vi "rsidr_core_global.vi"() -> ()   [LabVIEW 2020, in "Rohde&Schwarz RTx Oscilloscopes.lvlib"] (continued)
{"Level"=3, "Class Only"=FALSE, "Identifier"="RSRTX_ATTR_QUICK_MEASUREMENTS_DISABLE", "Descriptive Name"="Quick Measurements Disable", "Data Type"=4, "Command"="MEAS{Measurement}:AOFF", "Access"=1, "Range Table"="", "Read Callback"="", "Write Callback"="", "Supported Models"="", "Instrument Options"="", "Flags"=0, "Help"="Disables all additional measurements in all categories of the indicated measurement.\n\nAvailable Repeated Capabilities:\nMeasurement: M1, M2, M3, M4, M5, M6, M7, M8\r\n\nRemote-control command(s):\nMEASurement<m>:AOFF"}, {"Level"=3, "Class Only"=FALSE, "Identifier"="RSRTX_ATTR_QUICK_MEASUREMENTS_ENABLE_WITH_STATUS_BIT", "Descriptive Name"="Quick Measurements Enable With Status Bit", "Data Type"=3, "Command"="MEAS{Measurement}:ALL", "Access"=2, "Range Table"="", "Read Callback"="", "Write Callback"="", "Supported Models"="", "Instrument Options"="", "Flags"=0, "Help"="Enables and disables quick measurement.\n\nAvailable Repeated Capabilities:\nMeasurement: M1, M2, M3, M4, M5, M6, M7, M8\r\n\nRemote-control command(s):\nMEASurement<m>:ALL[:STATe]"}, {"Level"=2, "Class Only"=TRUE, "Identifier"="", "Descriptive Name"="Automatic Measurements - Statistics", "Data Type"=0, "Command"="", "Access"=0, "Range Table"="", "Read Callback"="", "Write Callback"="", "Supported Models"="", "Instrument Options"="", "Flags"=0, "Help"="Automatic Measurements - Statistics settings and results"}, {"Level"=3, "Class Only"=FALSE, "Identifier"="RSRTX_ATTR_AUTOMATIC_MEASUREMENT_ENABLED", "Descriptive Name"="Automatic Measurement Enabled", "Data Type"=3, "Command"="MEAS{Measurement}:STAT", "Access"=2, "Range Table"="", "Read Callback"="", "Write Callback"="", "Supported Models"="", "Instrument Options"="", "Flags"=0, "Help"="Activates or deactivates the statistical evaluation for the selected measurement.\n\nAvailable Repeated Capabilities:\nMeasurement: M1, M2, M3, M4, M5, M6, M7, M8\r\n\nRemote-control command(s):\nMEASurement<m>:STATistics[:ENABle]"}, {"Level"=3, "Class Only"=FALSE, "Identifier"="RSRTX_ATTR_AUTOMATIC_MEASUREMENT_NUMBER_OF_WAVEFORMS", "Descriptive Name"="Automatic Measurement Number Of Waveforms", "Data Type"=0, "Command"="MEAS{Measurement}:STAT:WEIG?", "Access"=0, "Range Table"="rsrtx_rngAutoMeasWaveforms", "Read Callback"="", "Write Callback"="", "Supported Models"="", "Instrument Options"="", "Flags"=0, "Help"="Returns the size of the statistics buffer. The buffer size is always 1000 result values.\n\nAvailable Repeated Capabilities:\nMeasurement: M1, M2, M3, M4, M5, M6, M7, M8\r\n\nRemote-control command(s):\nMEASurement<m>:STATistics:WEIGht?"}, {"Level"=3, "Class Only"=FALSE, "Identifier"="RSRTX_ATTR_RESET_AUTOMATIC_MEASUREMENT", "Descriptive Name"="Reset Automatic Measurement", "Data Type"=4, "Command"="MEAS{Measurement}:STAT:RES", "Access"=1, "Range Table"="", "Read Callback"="", "Write Callback"="", "Supported Models"="", "Instrument Options"="", "Flags"=0, "Help"="This attributedeletes the statistical results for the selected measurement, and starts a new statistical evaluation if the acquisition is running. The waveform count is set to 0 and all measurement values are set to NAN.\n\nAvailable Repeated Capabilities:\nMeasurement: M1, M2, M3, M4, M5, M6, M7, M8\r\n\nRemote-control command(s):\nMEASurement<m>:STATistics:RESet"}, {"Level"=3, "Class Only"=FALSE, "Identifier"="RSRTX_ATTR_AUTOMATIC_MEASUREMENT_NUMBER_OF_MEASURED_WAVEFORMS", "Descriptive Name"="Automatic Measurement Number Of Measured Waveforms", "Data Type"=0, "Command"="MEAS{Measurement}:RES:WFMC?", "Access"=0, "Range Table"="", "Read Callback"="", "Write Callback"="", "Supported Models"="", "Instrument Options"="", "Flags"=0, "Help"="Returns the current number of measured waveforms.\n\nAvailable Repeated Capabilities:\nMeasurement: M1, M2, M3, M4, M5, M6, M7, M8\r\n\nRemote-control command(s):\nMEASurement<m>:RESult:WFMCount?"}, {"Level"=3, "Class Only"=FALSE, "Identifier"="RSRTX_ATTR_AUTOMATIC_MEASUREMENT_TIMEOUT_AUTO", "Descriptive Name"="Automatic Measurement Timeout Auto", "Data Type"=3, "Command"="MEAS{Measurement}:TIM:AUTO", "Access"=2, "Range Table"="", "Read Callback"="", "Write Callback"="", "Supported Models"="", "Instrument Options"="", "Flags"=0, "Help"="The waiting time is set automatically, based on the horizontal scale.\n\nAvailable Repeated Capabilities:\nMeasurement: M1, M2, M3, M4, M5, M6, M7, M8\r\n\nRemote-control command(s):\nMEASurement<m>:TIMeout:AUTO"}, {"Level"=3, "Class Only"=FALSE, "Identifier"="RSRTX_ATTR_AUTOMATIC_MEASUREMENT_TIMEOUT", "Descriptive Name"="Automatic Measurement Timeout", "Data Type"=1, "Command"="MEAS{Measurement}:TIM", "Access"=2, "Range Table"="", "Read Callback"="", "Write Callback"="", "Supported Models"="", "Instrument Options"="", "Flags"=0, "Help"="Sets a waiting time, how long the instrument waits until it returns the measurement results.\n\nAvailable Repeated Capabilities:\nMeasurement: M1, M2, M3, M4, M5, M6, M7, M8\r\n\nRemote-control command(s):\nMEASurement<m>:TIMeout[TIME]"}, {"Level"=3, "Class Only"=FALSE, "Identifier"="RSRTX_ATTR_AUTOMATIC_MEASUREMENT_RESULT_AVERAGE_VALUE", "Descriptive Name"="Automatic Measurement Result Average Value", "Data Type"=1, "Command"="MEAS{Measurement}:RES:AVG?", "Access"=0, "Range Table"="", "Read Callback"="", "Write Callback"="", "Supported Models"="", "Instrument Options"="", "Flags"=0, "Help"="Returns the result of the automatic measurement.\n\nAvailable Repeated Capabilities:\nMeasurement: M1, M2, M3, M4, M5, M6, M7, M8\r\n\nRemote-control command(s):\nMEASurement<m>:RESult:AVG?"}, {"Level"=3, "Class Only"=FALSE, "Identifier"="RSRTX_ATTR_AUTOMATIC_MEASUREMENT_RESULT_STANDARD_DEVIATION", "Descriptive Name"="Automatic Measurement Result Standard Deviation", "Data Type"=1, "Command"="MEAS{Measurement}:RES:STDD?", "Access"=0, "Range Table"="", "Read Callback"="", "Write Callback"="", "Supported Models"="", "Instrument Options"="", "Flags"=0, "Help"="Returns the result of the automatic measurement.\n\nAvailable Repeated Capabilities:\nMeasurement: M1, M2, M3, M4, M5, M6, M7, M8\r\n\nRemote-control command(s):\nMEASurement<m>:RESult:STDDev?"}, {"Level"=3, "Class Only"=FALSE, "Identifier"="RSRTX_ATTR_AUTOMATIC_MEASUREMENT_RESULT_NEGATIVE_PEAK", "Descriptive Name"="Automatic Measurement Result Negative Peak", "Data Type"=1, "Command"="MEAS{Measurement}:RES:NPE?", "Access"=0, "Range Table"="", "Read Callback"="", "Write Callback"="", "Supported Models"="", "Instrument Options"="", "Flags"=0, "Help"="Returns the result of the automatic measurement.\n\nAvailable Repeated Capabilities:\nMeasurement: M1, M2, M3, M4, M5, M6, M7, M8\r\n\nRemote-control command(s):\nMEASurement<m>:RESult:NPEak?"}, {"Level"=3, "Class Only"=FALSE, "Identifier"="RSRTX_ATTR_AUTOMATIC_MEASUREMENT_RESULT_POSITIVE_PEAK", "Descriptive Name"="Automatic Measurement Result Positive Peak", "Data Type"=1, "Command"="MEAS{Measurement}:RES:PPE?", "Access"=0, "Range Table"="", "Read Callback"="", "Write Callback"="", "Supported Models"="", "Instrument Options"="", "Flags"=0, "Help"="Returns the result of the automatic measurement.\n\nAvailable Repeated Capabilities:\nMeasurement: M1, M2, M3, M4, M5, M6, M7, M8\r\n\nRemote-control command(s):\nMEASurement<m>:RESult:PPEak?"}, {"Level"=3, "Class Only"=FALSE, "Identifier"="RSRTX_ATTR_AUTOMATIC_MEASUREMENT_RESULT_INDEX", "Descriptive Name"="Automatic Measurement Result Index", "Data Type"=0, "Command"="", "Access"=2, "Range Table"="rsrtx_rngAutomaticMeasurementResultIndex", "Read Callback"="", "Write Callback"="", "Supported Models"="", "Instrument Options"="", "Flags"=0, "Help"="Selector for statistical result from RSRTX_ATTR_AUTOMATIC_MEASUREMENT_SINGLE_STATISTICAL_VALUE query.\n\nAvailable Repeated Capabilities:\nNone\n\nRemote-control command(s):\n"}, {"Level"=3, "Class Only"=FALSE, "Identifier"="RSRTX_ATTR_AUTOMATIC_MEASUREMENT_SINGLE_STATISTICAL_VALUE", "Descriptive Name"="Automatic Measurement Single Statistical Value", "Data Type"=1, "Command"="MEAS{Measurement}:STAT:VAL<Place>?", "Access"=0, "Range Table"="", "Read Callback"="rsrtx_singleStatisticalValue_ReadCallback.vi", "Write Callback"="", "Supported Models"="", "Instrument Options"="", "Flags"=2, "Help"="Returns one statistical value from the indicated buffer place. Place is indicated by value of RSRTX_ATTR_AUTOMATIC_MEASUREMENT_RESULT_INDEX attribute.\n\nAvailable Repeated Capabilities:\nMeasurement: M1, M2, M3, M4, M5, M6, M7, M8\r\n\nRemote-control command(s):\nMEASurement<m>:STATistics:VALue<n>?"}, {"Level"=3, "Class Only"=TRUE, "Identifier"="", "Descriptive Name"="Export Automatic Measurements", "Data Type"=0, "Command"="", "Access"=0, "Range Table"="", "Read Callback"="", "Write Callback"="", "Supported Models"="", "Instrument Options"="", "Flags"=0, "Help"="Contains attributes for Exporting the results to the CSV files."}, {"Level"=4, "Class Only"=FALSE, "Identifier"="RSRTX_ATTR_EXPORT_AUTOMATIC_MEASUREMENTS_NAME", "Descriptive Name"="Export Automatic Measurements Name", "Data Type"=2, "Command"="EXP:MEAS{Measurement}:STAT:NAME", "Access"=2, "Range Table"="", "Read Callback"="", "Write Callback"="", "Supported Models"="", "Instrument Options"="", "Flags"=0, "Help"="Defines the path and filename of the statistics file. The file format is CSV. If the file already exists, it will be overwritten.\n\nAvailable Repeated Capabilities:\nMeasurement: M1, M2, M3, M4, M5, M6, M7, M8\r\n\nRemote-control command(s):\nEXPort:MEASurement<m>:STATistics:NAME"}, {"Level"=4, "Class Only"=FALSE, "Identifier"="RSRTX_ATTR_EXPORT_AUTOMATIC_MEASUREMENT_SAVE", "Descriptive Name"="Export Automatic Measurement Save", "Data Type"=4, "Command"="EXP:MEAS{Measurement}:STAT:SAVE", "Access"=1, "Range Table"="", "Read Callback"="", "Write Callback"="", "Supported Models"="", "Instrument Options"="", "Flags"=0, "Help"="Saves statistical results of the indicated measurement place to the file that is defined by the EXPort:MEASurement<m>:STATistics:NAME command.\n\nAvailable Repeated Capabilities:\nMeasurement: M1, M2, M3, M4, M5, M6, M7, M8\r\n\nRemote-control command(s):\nEXPort:MEASurement<m>:STATistics:SAVE"}, {"Level"=4, "Class Only"=FALSE, "Identifier"="RSRTX_ATTR_EXPORT_AUTOMATIC_MEASUREMENTS_ALL_NAME", "Descriptive Name"="Export Automatic Measurements All Name", "Data Type"=2, "Command"="EXP:MEAS:STAT:ALL:NAME", "Access"=1, "Range Table"="", "Read Callback"="", "Write Callback"="", "Supported Models"="", "Instrument Options"="", "Flags"=0, "Help"="Defines the path and filename of the statistics file. The file format is CSV. If the file already exists, it will be overwritten.\n\nAvailable Repeated Capabilities:\nNone\n\nRemote-control command(s):\nEXPort:MEASurement:STATistics:ALL:NAME"}, {"Level"=4, "Class Only"=FALSE, "Identifier"="RSRTX_ATTR_EXPORT_AUTOMATIC_MEASUREMENT_ALL_SAVE", "Descriptive Name"="Export Automatic Measurement All Save", "Data Type"=4, "Command"="EXP:MEAS:STAT:ALL:SAVE", "Access"=1, "Range Table"="", "Read Callback"="", "Write Callback"="", "Supported Models"="", "Instrument Options"="", "Flags"=0, "Help"="Saves statistical results of the indicated measurement place to the file that is defined by RSRTX_ATTR_EXPORT_AUTOMATIC_MEASUREMENTS_ALL_NAME.\n\nAvailable Repeated Capabilities:\nNone\n\nRemote-control command(s):\nEXPort:MEASurement:STATistics:ALL:SAVE"}, {"Level"=2, "Class Only"=TRUE, "Identifier"="", "Descriptive Name"="Gate", "Data Type"=0, "Command"="", "Access"=0, "Range Table"="", "Read Callback"="", "Write Callback"="", "Supported Models"="", "Instrument Options"="", "Flags"=0, "Help"="This class contains methods for configuring the measurement gate."}, {"Level"=3, "Class Only"=FALSE, "Identifier"="RSRTX_ATTR_MEASUREMENT_GATE_ENABLE", "Descriptive Name"="Measurement Gate Enable", "Data Type"=3, "Command"="MEAS:GATE", "Access"=2, "Range Table"="", "Read Callback"="", "Write Callback"="", "Supported Models"="", "Instrument Options"="", "Flags"=0, "Help"="Activates or deactivates the measurement gate.\n\nAvailable Repeated Capabilities:\nNone\n\nRemote-control command(s):\nMEASurement<m>:GATE"}, {"Level"=3, "Class Only"=FALSE, "Identifier"="RSRTX_ATTR_MEASUREMENT_GATE_MODE", "Descriptive Name"="Measurement Gate Mode", "Data Type"=0, "Command"="MEAS:GATE:MODE", "Access"=2, "Range Table"="RsRtx_rngAbsoluteRelative", "Read Callback"="", "Write Callback"="", "Supported Models"="", "Instrument Options"="", "Flags"=0, "Help"="Defines whether the gate is defined in absolute or relative values.\n\nAvailable Repeated Capabilities:\nNone\n\nRemote-control command(s):\nMEASurement<m>:GATE:MODE"}, {"Level"=3, "Class Only"=FALSE, "Identifier"="RSRTX_ATTR_MEASUREMENT_GATE_ABSOLUTE_START", "Descriptive Name"="Measurement Gate Absolute Start", "Data Type"=1, "Command"="MEAS:GATE:ABS:STAR", "Access"=2, "Range Table"="", "Read Callback"="", "Write Callback"="", "Supported Models"="", "Instrument Options"="", "Flags"=0, "Help"="Defines the absolute start time for the measurement gate in seconds.\n\nAvailable Repeated Capabilities:\nNone\n\nRemote-control command(s):\nMEASurement<m>:GATE:ABSolute:STARt"}, {"Level"=3, "Class Only"=FALSE, "Identifier"="RSRTX_ATTR_MEASUREMENT_GATE_ABSOLUTE_END", "Descriptive Name"="Measurement Gate Absolute End", "Data Type"=1, "Command"="MEAS:GATE:ABS:STOP", "Access"=2, "Range Table"="", "Read Callback"="", "Write Callback"="", "Supported Models"="", "Instrument Options"="", "Flags"=0, "Help"="Defines the absolute end time for the measurement gate in seconds.\n\nAvailable Repeated Capabilities:\nNone\n\nRemote-control command(s):\nMEASurement<m>:GATE:ABSolute:STOP"}, {"Level"=3, "Class Only"=FALSE, "Identifier"="RSRTX_ATTR_MEASUREMENT_GATE_RELATIVE_START", "Descriptive Name"="Measurement Gate Relative Start", "Data Type"=1, "Command"="MEAS:GATE:REL:STAR", "Access"=2, "Range Table"="", "Read Callback"="", "Write Callback"="", "Supported Models"="", "Instrument Options"="", "Flags"=0, "Help"="Defines the relative start value for the measurement gate in %.\n\nAvailable Repeated Capabilities:\nNone\n\nRemote-control command(s):\nMEASurement<m>:GATE:RELative:STARt"}, {"Level"=3, "Class Only"=FALSE, "Identifier"="RSRTX_ATTR_MEASUREMENT_GATE_RELATIVE_END", "Descriptive Name"="Measurement Gate Relative End", "Data Type"=1, "Command"="MEAS:GATE:REL:STOP", "Access"=2, "Range Table"="", "Read Callback"="", "Write Callback"="", "Supported Models"="", "Instrument Options"="", "Flags"=0, "Help"="Defines the relative end value for the measurement gate in %.\n\nAvailable Repeated Capabilities:\nNone\n\nRemote-control command(s):\nMEASurement<m>:GATE:RELative:STOP"}, {"Level"=1, "Class Only"=TRUE, "Identifier"="", "Descriptive Name"="Mathematics", "Data Type"=0, "Command"="", "Access"=0, "Range Table"="", "Read Callback"="", "Write Callback"="", "Supported Models"="", "Instrument Options"="", "Flags"=0, "Help"="The instrument provides different methods of creating mathematical waveforms:\n- Applying mathematical functions to source data\n- Performing FFT analysis on source data"}, {"Level"=2, "Class Only"=FALSE, "Identifier"="RSRTX_ATTR_MATH_WAVEFORM_HEADER", "Descriptive Name"="Math Waveform Header", "Data Type"=2, "Command"="CALC:MATH{Math}:DATA:HEAD?", "Access"=0, "Range Table"="", "Read Callback"="", "Write Callback"="", "Supported Models"="RTM|RTA", "Instrument Options"="", "Flags"=0, "Help"="Returns the header of math waveform data. The header contains attributes of the waveform.\n\nAvailable Repeated Capabilities:\nMath: MA1, MA2, MA3, MA4, MA5\r\n\nRemote-control command(s):\nCALCulate:MATH<m>:DATA:HEADer?"}, {"Level"=2, "Class Only"=FALSE, "Identifier"="RSRTX_ATTR_MATH_WAVEFORM_DATA_POINTS", "Descriptive Name"="Math Waveform Data Points", "Data Type"=0, "Command"="CALC:MATH{Math}:DATA:POIN?", "Access"=0, "Range Table"="", "Read Callback"="", "Write Callback"="", "Supported Models"="RTM|RTA", "Instrument Options"="", "Flags"=0, "Help"="Returns the number of data samples that are returned with CALCulate:MATH<m>:DATA?.\n\nAvailable Repeated Capabilities:\nMath: MA1, MA2, MA3, MA4, MA5\r\n\nRemote-control command(s):\nCALCulate:MATH<m>:DATA:POINts?"}, {"Level"=2, "Class Only"=TRUE, "Identifier"="", "Descriptive Name"="Mathematics General", "Data Type"=0, "Command"="", "Access"=0, "Range Table"="", "Read Callback"="", "Write Callback"="", "Supported Models"="", "Instrument Options"="", "Flags"=0, "Help"="General mathematics parameters."}, {"Level"=3, "Class Only"=FALSE, "Identifier"="RSRTX_ATTR_MATH_WAVEFORM_ENABLED", "Descriptive Name"="Math Waveform Enabled", "Data Type"=3, "Command"="CALC:MATH{Math}:STAT", "Access"=2, "Range Table"="", "Read Callback"="", "Write Callback"="", "Supported Models"="RTM|RTA", "Instrument Options"="", "Flags"=0, "Help"="Enables the math waveform display.\n\nAvailable Repeated Capabilities:\nMath: MA1, MA2, MA3, MA4, MA5\r\n\nRemote-control command(s):\nCALCulate:MATH<m>:STATe"}, {"Level"=3, "Class Only"=FALSE, "Identifier"="RSRTX_ATTR_MATH_WAVEFORM_POSITION", "Descriptive Name"="Math Waveform Position", "Data Type"=1, "Command"="CALC:MATH{Math}:POS", "Access"=2, "Range Table"="rsrtx_rngWaveformPosition", "Read Callback"="", "Write Callback"="", "Supported Models"="RTM|RTA", "Instrument Options"="", "Flags"=0, "Help"="Sets the vertical position of the specified math waveform in the window.\n\nAvailable Repeated Capabilities:\nMath: MA1, MA2, MA3, MA4, MA5\r\n\nRemote-control command(s):\nCALCulate:MATH<m>:POSition"}, {"Level"=3, "Class Only"=FALSE, "Identifier"="RSRTX_ATTR_MATH_VERTICAL_SCALE", "Descriptive Name"="Math Vertical Scale", "Data Type"=1, "Command"="CALC:MATH{Math}:SCAL", "Access"=2, "Range Table"="rsrtx_rngMathVerticalScale", "Read Callback"="", "Write Callback"="", "Supported Models"="RTM|RTA", "Instrument Options"="", "Flags"=0, "Help"="Sets the vertical position of the specified math waveform in the window.\n\nAvailable Repeated Capabilities:\nMath: MA1, MA2, MA3, MA4, MA5\r\n\nRemote-control command(s):\nCALCulate:MATH<m>:SCALe"}, {"Level"=3, "Class Only"=FALSE, "Identifier"="RSRTX_ATTR_MATH_ACQUISITION_TYPE", "Descriptive Name"="Math Acquisition Type", "Data Type"=0, "Command"="CALC:MATH{Math}:ARIT", "Access"=2, "Range Table"="rsrtx_rngWaveformArithmetics", "Read Callback"="", "Write Callback"="", "Supported Models"="RTM|RTA", "Instrument Options"="", "Flags"=0, "Help"="Selects the method to build the resulting math waveform from consecutive acquisitions. The processing is similar to the waveform arithmetics - instead of the acquired waveforms the math waveforms are used to create envelope and average.\n\nAvailable Repeated Capabilities:\nMath: MA1, MA2, MA3, MA4, MA5\r\n\nRemote-control command(s):\nCALCulate:MATH<m>:ARIThmetics"}, {"Level"=3, "Class Only"=FALSE, "Identifier"="RSRTX_ATTR_MATH_EXPRESSION", "Descriptive Name"="Math Expression", "Data Type"=2, "Command"="CALC:MATH{Math}", "Access"=2, "Range Table"="", "Read Callback"="", "Write Callback"="", "Supported Models"="RTM|RTA", "Instrument Options"="", "Flags"=0, "Help"="Defines the math expression to be calculated for the specified math channel.\n\nAvailable Repeated Capabilities:\nMath: MA1, MA2, MA3, MA4, MA5\r\n\nRemote-control command(s):\nCALCulate:MATH<m>[:EXPRession][:DEFine]"}, {"Level"=3, "Class Only"=FALSE, "Identifier"="RSRTX_ATTR_MATH_WAVEFORM_LABEL", "Descriptive Name"="Math Waveform Label", "Data Type"=2, "Command"="CALC:MATH{Math}:LAB", "Access"=2, "Range Table"="", "Read Callback"="", "Write Callback"="", "Supported Models"="", "Instrument Options"="", "Flags"=0, "Help"="Defines a label for the specified math waveform (equation), which is shown at the waveform.\n\nAvailable Repeated Capabilities:\nMath: MA1, MA2, MA3, MA4, MA5\r\n\nRemote-control command(s):\nCALCulate:MATH<m>:LABel"}, {"Level"=3, "Class Only"=FALSE, "Identifier"="RSRTX_ATTR_MATH_WAVEFORM_LABEL_STATE", "Descriptive Name"="Math Waveform Label State", "Data Type"=3, "Command"="CALC:MATH{Math}:LAB:STAT", "Access"=2, "Range Table"="", "Read Callback"="", "Write Callback"="", "Supported Models"="", "Instrument Options"="", "Flags"=0, "Help"="Activates the diplay of the label that is defined with RSRTX_ATTR_MATH_WAVEFORM_LABEL.\n\nAvailable Repeated Capabilities:\nMath: MA1, MA2, MA3, MA4, MA5\r\n\nRemote-control command(s):\nCALCulate:MATH<m>:LABel:STATe"}, {"Level"=3, "Class Only"=FALSE, "Identifier"="RSRTX_ATTR_MATH_WAVEFORM_COLOR", "Descriptive Name"="Math Waveform Color", "Data Type"=0, "Command"="CALC:MATH{Math}:WCOL", "Access"=2, "Range Table"="RsRtx_rngMathWaveformColor", "Read Callback"="", "Write Callback"="", "Supported Models"="", "Instrument Options"="", "Flags"=0, "Help"="Sets the color of the indicated math waveform.\n\nAvailable Repeated Capabilities:\nMath: MA1, MA2, MA3, MA4, MA5\r\n\nRemote-control command(s):\nCALCulate:MATH<m>:WCOLor"}, {"Level"=2, "Class Only"=TRUE, "Identifier"="", "Descriptive Name"="Mathematics FFT", "Data Type"=0, "Command"="", "Access"=0, "Range Table"="", "Read Callback"="", "Write Callback"="", "Supported Models"="", "Instrument Options"="", "Flags"=0, "Help"="Attributes for setting FFT parameters. During FFT analysis, a signal in the time domain is  converted to a spectrum of frequencies. A basic FFT waveform can be displayed very quickly. By defining additional FFT parameters, the waveform can be configured in more detail. As a result, either the magnitude or the phase of the determined frequencies can be displayed, or more complex FFT functions. Analysis can be restricted to an extract of the original time base, and the results display can be restricted to a specified frequency range."}, {"Level"=3, "Class Only"=FALSE, "Identifier"="RSRTX_ATTR_FFT_CENTER_FREQUENCY", "Descriptive Name"="FFT Center Frequency", "Data Type"=1, "Command"="CALC:MATH{Math}:FFT:CFR", "Access"=2, "Range Table"="", "Read Callback"="", "Write Callback"="", "Supported Models"="", "Instrument Options"="", "Flags"=0, "Help"="Defines the position of the displayed frequency range, which is (Center - Span/2) to (Center + Span/2).\n\nAvailable Repeated Capabilities:\nMath: MA1, MA2, MA3, MA4, MA5\r\n\nRemote-control command(s):\nCALCulate:MATH<m>:FFT:CFRequency"}, {"Level"=3, "Class Only"=FALSE, "Identifier"="RSRTX_ATTR_FFT_FREQUENCY_SPAN", "Descriptive Name"="FFT Frequency Span", "Data Type"=1, "Command"="CALC:MATH{Math}:FFT:SPAN", "Access"=2, "Range Table"="", "Read Callback"="", "Write Callback"="", "Supported Models"="", "Instrument Options"="", "Flags"=0, "Help"="The span is specified in Hertz and defines the width of the displayed frequency range, which is (Center - Span/2) to (Center + Span/2).\n\nAvailable Repeated Capabilities:\nMath: MA1, MA2, MA3, MA4, MA5\r\n\nRemote-control command(s):\nCALCulate:MATH<m>:FFT:SPAN"}, {"Level"=3, "Class Only"=FALSE, "Identifier"="RSRTX_ATTR_FFT_FULL_SPAN", "Descriptive Name"="FFT Full Span", "Data Type"=4, "Command"="CALC:MATH{Math}:FFT:FULL", "Access"=1, "Range Table"="", "Read Callback"="", "Write Callback"="", "Supported Models"="", "Instrument Options"="", "Flags"=0, "Help"="Performs FFT calculation for the full frequency span.\n\nAvailable Repeated Capabilities:\nMath: MA1, MA2, MA3, MA4, MA5\r\n\nRemote-control command(s):\nCALCulate:MATH<m>:FFT:FULLspan"}, {"Level"=3, "Class Only"=FALSE, "Identifier"="RSRTX_ATTR_FFT_START_FREQUENCY", "Descriptive Name"="FFT Start Frequency", "Data Type"=1, "Command"="CALC:MATH{Math}:FFT:STAR", "Access"=2, "Range Table"="", "Read Callback"="", "Write Callback"="", "Supported Models"="", "Instrument Options"="", "Flags"=0, "Help"="Defines the start frequency of the displayed frequency span.\n\nAvailable Repeated Capabilities:\nMath: MA1, MA2, MA3, MA4, MA5\r\n\nRemote-control command(s):\nCALCulate:MATH<m>:FFT:STARt"}, {"Level"=3, "Class Only"=FALSE, "Identifier"="RSRTX_ATTR_FFT_STOP_FREQUENCY", "Descriptive Name"="FFT Stop Frequency", "Data Type"=1, "Command"="CALC:MATH{Math}:FFT:STOP", "Access"=2, "Range Table"="", "Read Callback"="", "Write Callback"="", "Supported Models"="", "Instrument Options"="", "Flags"=0, "Help"="Defines the stop frequency of the displayed frequency span.\n\nAvailable Repeated Capabilities:\nMath: MA1, MA2, MA3, MA4, MA5\r\n\nRemote-control command(s):\nCALCulate:MATH<m>:FFT:STOP"}, {"Level"=3, "Class Only"=FALSE, "Identifier"="RSRTX_ATTR_FFT_AVERAGING", "Descriptive Name"="FFT Averaging", "Data Type"=0, "Command"="CALC:MATH{Math}:FFT:AVER:COUN", "Access"=2, "Range Table"="rsrtx_rngAveragingSpectrums", "Read Callback"="", "Write Callback"="", "Supported Models"="", "Instrument Options"="", "Flags"=0, "Help"="Defines the number of spectrums used for averaging if CALCulate: MATH<m>:ARIThmetics is set to AVERage.\n\nAvailable Repeated Capabilities:\nMath: MA1, MA2, MA3, MA4, MA5\r\n\nRemote-control command(s):\nCALCulate:MATH<m>:FFT:AVERage:COUNt"}, {"Level"=3, "Class Only"=FALSE, "Identifier"="RSRTX_ATTR_FFT_AVERAGING_STATUS", "Descriptive Name"="FFT Averaging Status", "Data Type"=3, "Command"="CALC:MATH{Math}:FFT:AVER:COMP?", "Access"=0, "Range Table"="", "Read Callback"="", "Write Callback"="", "Supported Models"="", "Instrument Options"="", "Flags"=0, "Help"="Returns the state of spectrum averaging.\nFalse - The number of acquired waveforms is less than the number required for average calculation. See RSRTX_ATTR_FFT_AVERAGING.\nTrue - The instrument acquired a sufficient number of waveforms to determine the average.\n\nAvailable Repeated Capabilities:\nMath: MA1, MA2, MA3, MA4, MA5\r\n\nRemote-control command(s):\nCALCulate:MATH<m>:FFT:AVERage:COMPlete?"}, {"Level"=3, "Class Only"=FALSE, "Identifier"="RSRTX_ATTR_FFT_WINDOW_TYPE", "Descriptive Name"="FFT Window Type", "Data Type"=0, "Command"="CALC:MATH{Math}:FFT:WIND:TYPE", "Access"=2, "Range Table"="rsrtx_rngFFTWindowType", "Read Callback"="", "Write Callback"="", "Supported Models"="", "Instrument Options"="", "Flags"=0, "Help"="Windowing helps minimize the discontinuities at the end of the measured signal interval and thus reduces the effect of spectral leakage, increasing the frequency resolution.\nVarious different window functions are provided to suit different input signals. Each of the window functions has specific characteristics, including some advantages and some trade-offs. These characteristics need to be considered carefully to find the optimum solution for the measurement task.\n\nAvailable Repeated Capabilities:\nMath: MA1, MA2, MA3, MA4, MA5\r\n\nRemote-control command(s):\nCALCulate:MATH<m>:FFT:WINDow:TYPE"}, {"Level"=3, "Class Only"=FALSE, "Identifier"="RSRTX_ATTR_FFT_RESOLUTION_BANDWIDTH", "Descriptive Name"="FFT Resolution Bandwidth", "Data Type"=1, "Command"="CALC:MATH{Math}:FFT:BAND", "Access"=2, "Range Table"="rsrtx_rngRBW", "Read Callback"="", "Write Callback"="", "Supported Models"="", "Instrument Options"="", "Flags"=0, "Help"="Defines the resolution bandwidth.\n\nAvailable Repeated Capabilities:\nMath: MA1, MA2, MA3, MA4, MA5\r\n\nRemote-control command(s):\nCALCulate:MATH<m>:FFT:BANDwidth[:RESolution][:VALue]"}, {"Level"=3, "Class Only"=FALSE, "Identifier"="RSRTX_ATTR_FFT_RESOLUTION_BANDWIDTH_COUPLING_ENABLED", "Descriptive Name"="FFT Resolution Bandwidth Coupling Enabled", "Data Type"=3, "Command"="CALC:MATH{Math}:FFT:BAND:AUTO", "Access"=2, "Range Table"="", "Read Callback"="", "Write Callback"="", "Supported Models"="", "Instrument Options"="", "Flags"=0, "Help"="Couples the frequency span to the RBW.\n\nAvailable Repeated Capabilities:\nMath: MA1, MA2, MA3, MA4, MA5\r\n\nRemote-control command(s):\nCALCulate:MATH<m>:FFT:BANDwidth[:RESolution]:AUTO"}, {"Level"=3, "Class Only"=FALSE, "Identifier"="RSRTX_ATTR_FFT_RESOLUTION_BANDWIDTH_RATIO", "Descriptive Name"="FFT Resolution Bandwidth Ratio", "Data Type"=1, "Command"="CALC:MATH{Math}:FFT:BAND:RAT", "Access"=2, "Range Table"="rsrtx_rngRBWRatio", "Read Callback"="", "Write Callback"="", "Supported Models"="", "Instrument Options"="", "Flags"=0, "Help"="Defines the ratio resolution bandwidth (Hz) / span (Hz).\n\nAvailable Repeated Capabilities:\nMath: MA1, MA2, MA3, MA4, MA5\r\n\nRemote-control command(s):\nCALCulate:MATH<m>:FFT:BANDwidth[:RESolution]:RATio"}, {"Level"=3, "Class Only"=FALSE, "Identifier"="RSRTX_ATTR_FFT_EFFECTIVE_RESOLUTION_BANDWIDTH", "Descriptive Name"="FFT Effective Resolution Bandwidth", "Data Type"=1, "Command"="CALC:MATH{Math}:FFT:BAND:ADJ?", "Access"=0, "Range Table"="", "Read Callback"="", "Write Callback"="", "Supported Models"="", "Instrument Options"="", "Flags"=0, "Help"="Queries the effective resolution bandwidth.\n\nAvailable Repeated Capabilities:\nMath: MA1, MA2, MA3, MA4, MA5\r\n\nRemote-control command(s):\nCALCulate:MATH<m>:FFT:BANDwidth[:RESolution]:ADJusted?"}, {"Level"=3, "Class Only"=FALSE, "Identifier"="RSRTX_ATTR_FFT_SCALING_UNIT", "Descriptive Name"="FFT Scaling Unit", "Data Type"=0, "Command"="CALC:MATH{Math}:FFT:MAGN:SCAL", "Access"=2, "Range Table"="rsrtx_rngScalingUnit", "Read Callback"="", "Write Callback"="", "Supported Models"="", "Instrument Options"="", "Flags"=0, "Help"="efines the scaling unit of the y-axis.\n\nAvailable Repeated Capabilities:\nMath: MA1, MA2, MA3, MA4, MA5\r\n\nRemote-control command(s):\nCALCulate:MATH<m>:FFT:MAGNitude:SCALe"}, {"Level"=3, "Class Only"=FALSE, "Identifier"="RSRTX_ATTR_FFT_SAMPLE_RATE", "Descriptive Name"="FFT Sample Rate", "Data Type"=1, "Command"="CALC:MATH{Math}:FFT:SRAT?", "Access"=0, "Range Table"="", "Read Callback"="", "Write Callback"="", "Supported Models"="", "Instrument Options"="", "Flags"=0, "Help"="Queries the sample rate of data used in an FFT analysis.\n\nAvailable Repeated Capabilities:\nMath: MA1, MA2, MA3, MA4, MA5\r\n\nRemote-control command(s):\nCALCulate:MATH<m>:FFT:SRATe?"}, {"Level"=3, "Class Only"=FALSE, "Identifier"="RSRTX_ATTR_FFT_YT_WINDOW_POSITION", "Descriptive Name"="FFT Yt Window Position", "Data Type"=1, "Command"="CALC:MATH{Math}:FFT:TIME:POS", "Access"=2, "Range Table"="", "Read Callback"="", "Write Callback"="", "Supported Models"="", "Instrument Options"="", "Flags"=0, "Help"="Sets the position of the time base extract in the Y(t)-window for which the FFT is calculated.\n\nAvailable Repeated Capabilities:\nMath: MA1, MA2, MA3, MA4, MA5\r\n\nRemote-control command(s):\nCALCulate:MATH<m>:FFT:TIME:POSition"}, {"Level"=3, "Class Only"=FALSE, "Identifier"="RSRTX_ATTR_FFT_YT_WINDOW_WIDTH", "Descriptive Name"="FFT Yt Window Width", "Data Type"=1, "Command"="CALC:MATH{Math}:FFT:TIME:RANG", "Access"=2, "Range Table"="", "Read Callback"="", "Write Callback"="", "Supported Models"="", "Instrument Options"="", "Flags"=0, "Help"="Sets the width of the time base extract from the Y(t)-window for which the FFT is calculated.\n\nAvailable Repeated Capabilities:\nMath: MA1, MA2, MA3, MA4, MA5\r\n\nRemote-control command(s):\nCALCulate:MATH<m>:FFT:TIME:RANGe"}, {"Level"=2, "Class Only"=TRUE, "Identifier"="", "Descriptive Name"="Mathematics Tracks", "Data Type"=0, "Command"="", "Access"=0, "Range Table"="", "Read Callback"="", "Write Callback"="", "Supported Models"="", "Instrument Options"="", "Flags"=0, "Help"="This class contains methods and attributes for mathematics on tracks. Math tracks are independent of the measurement functions. Bipolar signals have negative and positive pulses, unipolar signals have only positive pulses."}, {"Level"=3, "Class Only"=FALSE, "Identifier"="RSRTX_ATTR_MATH_TRACK_EDGE_POLARITY", "Descriptive Name"="Math Track Edge Polarity", "Data Type"=3, "Command"="CALC:MATH{Math}:TRAC:EDGE", "Access"=2, "Range Table"="", "Read Callback"="", "Write Callback"="", "Supported Models"="", "Instrument Options"="", "Flags"=0, "Help"="Sets the rising or falling edge as a reference for each measurement. The setting helps to determine values in terms of the power stage switching state. For unipolar souces, the on edge is the rising edge, and the off edge is the falling edge. In the bipolar case, all transitions are inverted for the negative branch. For positive pulses, the rising edge is the on edge, and for negative pulses, the falling edge is the on edge.\n\nAvailable Repeated Capabilities:\nMath: MA1, MA2, MA3, MA4, MA5\r\n\nRemote-control command(s):\nCALCulate:MATH<m>:TRACk:EDGE"}, {"Level"=3, "Class Only"=FALSE, "Identifier"="RSRTX_ATTR_MATH_TRACK_DOUBLE_PULSE_ENABLE", "Descriptive Name"="Math Track Double Pulse Enable", "Data Type"=3, "Command"="CALC:MATH{Math}:TRAC:DPUL", "Access"=2, "Range Table"="", "Read Callback"="", "Write Callback"="", "Supported Models"="", "Instrument Options"="", "Flags"=0, "Help"="Available for bipolar signals. Considers the effect of the double pulse, which arises due to the inversion.\n\nAvailable Repeated Capabilities:\nMath: MA1, MA2, MA3, MA4, MA5\r\n\nRemote-control command(s):\nCALCulate:MATH<m>:TRACk:DPULse[:ENABle]"}, {"Level"=3, "Class Only"=FALSE, "Identifier"="RSRTX_ATTR_MATH_TRACK_THRESHOLD_HYSTERESIS", "Descriptive Name"="Math Track Threshold Hysteresis", "Data Type"=1, "Command"="CALC:MATH{Math}:TRAC:THR:HYST", "Access"=2, "Range Table"="", "Read Callback"="", "Write Callback"="", "Supported Models"="", "Instrument Options"="", "Flags"=0, "Help"="Sets the hysteresis for correct edge detection.\n\nAvailable Repeated Capabilities:\nMath: MA1, MA2, MA3, MA4, MA5\r\n\nRemote-control command(s):\nCALCulate:MATH<m>:TRACk:THReshold:HYSTeresis"}, {"Level"=3, "Class Only"=FALSE, "Identifier"="RSRTX_ATTR_MATH_TRACK_THRESHOLD_LOWER", "Descriptive Name"="Math Track Threshold Lower", "Data Type"=1, "Command"="CALC:MATH{Math}:TRAC:THR:LOW", "Access"=2, "Range Table"="", "Read Callback"="", "Write Callback"="", "Supported Models"="", "Instrument Options"="", "Flags"=0, "Help"="Sets the lower level for bipolar track sources, which determines the crossing points on negative pulses.\n\nAvailable Repeated Capabilities:\nMath: MA1, MA2, MA3, MA4, MA5\r\n\nRemote-control command(s):\nCALCulate:MATH<m>:TRACk:THReshold:LOWer"}, {"Level"=3, "Class Only"=FALSE, "Identifier"="RSRTX_ATTR_MATH_TRACK_THRESHOLD_UPPER", "Descriptive Name"="Math Track Threshold Upper", "Data Type"=1, "Command"="CALC:MATH{Math}:TRAC:THR", "Access"=2, "Range Table"="", "Read Callback"="", "Write Callback"="", "Supported Models"="", "Instrument Options"="", "Flags"=0, "Help"="Sets the threshold for unipolar track sources, or the upper level for bipolar sources. The signal is measured at the crossing points of the signal with the threshold.\n\nAvailable Repeated Capabilities:\nMath: MA1, MA2, MA3, MA4, MA5\r\n\nRemote-control command(s):\nCALCulate:MATH<m>:TRACk:THReshold[:UPPer]"}, {"Level"=1, "Class Only"=TRUE, "Identifier"="", "Descriptive Name"="Simple Mathematics (RTB)", "Data Type"=0, "Command"="", "Access"=0, "Range Table"="", "Read Callback"="", "Write Callback"="", "Supported Models"="", "Instrument Options"="", "Flags"=0, "Help"="This class provides different methods of creating mathematical waveforms:\n- Applying mathematical functions to source data\n- Performing FFT analysis on source data"}, {"Level"=2, "Class Only"=FALSE, "Identifier"="RSRTX_ATTR_SIMPLE_MATH_WAVEFORM_ENABLED", "Descriptive Name"="Simple Math Waveform Enabled", "Data Type"=3, "Command"="CALC:QMATH:STAT", "Access"=2, "Range Table"="", "Read Callback"="", "Write Callback"="", "Supported Models"="RTB", "Instrument Options"="", "Flags"=0, "Help"="Activates the mathematics function and displays the resulting math waveform.\n\nAvailable Repeated Capabilities:\nNone\n\nRemote-control command(s):\nCALCulate:QMATH:STATe"}, {"Level"=2, "Class Only"=FALSE, "Identifier"="RSRTX_ATTR_SIMPLE_MATH_WAVEFORM_POSITION", "Descriptive Name"="Simple Math Waveform Position", "Data Type"=1, "Command"="CALC:QMAT:POS", "Access"=2, "Range Table"="", "Read Callback"="", "Write Callback"="", "Supported Models"="RTB", "Instrument Options"="", "Flags"=0, "Help"="Sets the vertical position of the math waveform.\n\nAvailable Repeated Capabilities:\nNone\n\nRemote-control command(s):\nCALCulate:QMATh:POSition"}, {"Level"=2, "Class Only"=FALSE, "Identifier"="RSRTX_ATTR_SIMPLE_MATH_WAVEFORM_VERTICAL_SCALE", "Descriptive Name"="Simple Math Waveform Vertical Scale", "Data Type"=1, "Command"="CALC:QMAT:SCAL", "Access"=2, "Range Table"="", "Read Callback"="", "Write Callback"="", "Supported Models"="RTB", "Instrument Options"="", "Flags"=0, "Help"="Sets the vertical scale of the math waveform.\n\nAvailable Repeated Capabilities:\nNone\n\nRemote-control command(s):\nCALCulate:QMATh:SCALe"}, {"Level"=2, "Class Only"=FALSE, "Identifier"="RSRTX_ATTR_SIMPLE_MATH_WAVEFORM_OPERATION", "Descriptive Name"="Simple Math Waveform Operation", "Data Type"=0, "Command"="CALC:QMAT:OPER", "Access"=2, "Range Table"="RsRtx_rngMathOperation", "Read Callback"="", "Write Callback"="", "Supported Models"="RTB", "Instrument Options"="", "Flags"=0, "Help"="Defines the operation that calculates the math waveform.\n\nAvailable Repeated Capabilities:\nNone\n\nRemote-control command(s):\nCALCulate:QMATh:OPERation"}, {"Level"=2, "Class Only"=TRUE, "Identifier"="", "Descriptive Name"="Source", "Data Type"=0, "Command"="", "Access"=0, "Range Table"="", "Read Callback"="", "Write Callback"="", "Supported Models"="", "Instrument Options"="", "Flags"=0, "Help"="Class for SourceNumber repcap."}, {"Level"=3, "Class Only"=FALSE, "Identifier"="RSRTX_ATTR_SIMPLE_MATH_WAVEFORM_SOURCE", "Descriptive Name"="Simple Math Waveform Source", "Data Type"=0, "Command"="CALC:QMAT:SOUR{SourceNumber}", "Access"=2, "Range Table"="rsrtx_rngMathSource", "Read Callback"="", "Write Callback"="", "Supported Models"="RTB", "Instrument Options"="", "Flags"=0, "Help"="Defines the first and the second source for the mathematical operation (operands). The sources can be any active analog channel.\n\nAvailable Repeated Capabilities:\nSourceNumber: S1, S2, S3, S4\r\n\nRemote-control command(s):\nCALCulate:QMATh:SOURce<m>"}, {"Level"=1, "Class Only"=TRUE, "Identifier"="", "Descriptive Name"="Reference Waveforms", "Data Type"=0, "Command"="", "Access"=0, "Range Table"="", "Read Callback"="", "Write Callback"="", "Supported Models"="", "Instrument Options"="", "Flags"=0, "Help"="Contains attributes for Reference Waveforms."}, {"Level"=2, "Class Only"=FALSE, "Identifier"="RSRTX_ATTR_REFERENCE_WAVEFORM_HEADER", "Descriptive Name"="Reference Waveform Header", "Data Type"=2, "Command"="REFC{ReferenceWfm}:DATA:HEAD?", "Access"=0, "Range Table"="", "Read Callback"="", "Write Callback"="", "Supported Models"="", "Instrument Options"="", "Flags"=0, "Help"="Returns information on the reference waveform.\n\nAvailable Repeated Capabilities:\nReferenceWfm: RW1, RW2, RW3, RW4\r\n\nRemote-control command(s):\nREFCurve<m>:DATA:HEADer?"}, {"Level"=2, "Class Only"=FALSE, "Identifier"="RSRTX_ATTR_REFERENCE_WAVEFORM_DATA_POINTS", "Descriptive Name"="Reference Waveform Data Points", "Data Type"=0, "Command"="REFC{ReferenceWfm}:DATA:POIN?", "Access"=0, "Range Table"="", "Read Callback"="", "Write Callback"="", "Supported Models"="", "Instrument Options"="", "Flags"=0, "Help"="Returns the number of data samples that are returned with REFCurve<m>:DATA?.\n\nAvailable Repeated Capabilities:\nReferenceWfm: RW1, RW2, RW3, RW4\r\n\nRemote-control command(s):\nREFCurve<m>:DATA:POINts?"}, {"Level"=2, "Class Only"=FALSE, "Identifier"="RSRTX_ATTR_REFERENCE_WAVEFORM_LABEL", "Descriptive Name"="Reference Waveform Label", "Data Type"=2, "Command"="REFC{ReferenceWfm}:LAB", "Access"=2, "Range Table"="", "Read Callback"="", "Write Callback"="", "Supported Models"="", "Instrument Options"="", "Flags"=0, "Help"="Defines a label for the indicated reference waveform.\n\nAvailable Repeated Capabilities:\nReferenceWfm: RW1, RW2, RW3, RW4\r\n\nRemote-control command(s):\nREFCurve<m>:LABel"}, {"Level"=2, "Class Only"=FALSE, "Identifier"="RSRTX_ATTR_REFERENCE_WAVEFORM_COLOR", "Descriptive Name"="Reference Waveform Color", "Data Type"=0, "Command"="REFC{ReferenceWfm}:WCOL", "Access"=2, "Range Table"="RsRtx_rngReferenceWaveformColor", "Read Callback"="", "Write Callback"="", "Supported Models"="", "Instrument Options"="", "Flags"=0, "Help"="Selects a color for the reference waveform. The default color
